vi "Write Multiple Coils.vi"(8 "error in":errorcluster, 9 "coils":bool[](array[boolean]), 10 "starting address":u16, 11 "device data model in":refnum<class "Standard Data Model.lvclass">) -> (0 "error out":errorcluster, 3 "device data model out":refnum<class "Standard Data Model.lvclass">)   [LabVIEW 2013, in "Modbus Library - Advance.lvlib" / "Standard Data Model.lvclass"]
doc: "Writes the values of multiple coils in series, starting at address M."
uses:
  Standard Data Model.lvclass
  Standard Data Model.lvclass/Standard Data Model.ctl
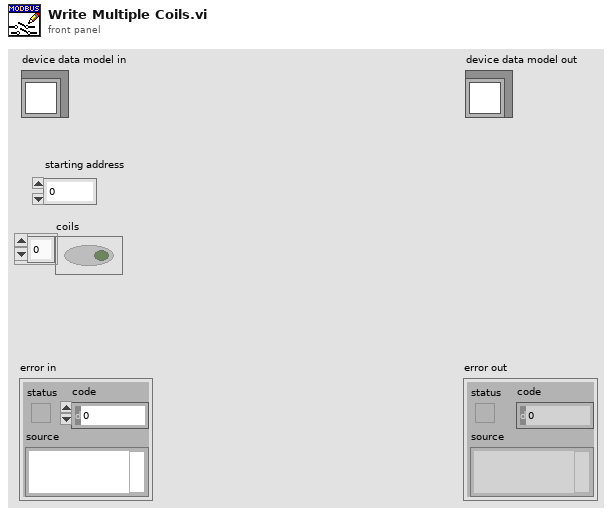
[diagram p1: front panel]
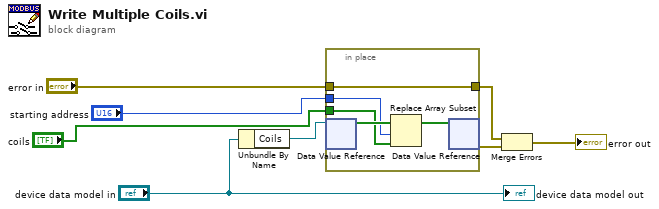
[diagram p0: block diagram]
diagram:
  n1 = Unbundle By Name("device data model in") -> ("Coils"=w5:refnum<data-value>)
  n2 = in-place {
    in-place-border: "error in" -> [w12]
    in-place-border: [w12] -> w3
    in-place-border: "starting address" -> [w10]
    in-place-border: "coils" -> [w9]
    n3 = in-place-dvr #1(w5) -> (w13:bool[])  [unwired: 1 out]
    n4 = Replace Array Subset(array=w13, new element=w9, index=w10) -> (w11:bool[])
    n5 = in-place-dvr #1(w11) -> (w4:errorcluster)  [unwired: 1 out]
  }
  n6 = Merge Errors(w3, w4) -> (→"error out":errorcluster)
  "device data model out" <- "device data model in"
